vi "Multidimensional Array Example.vi"() -> ()   [LabVIEW 2015, in "MsgPack.lvlib"]
uses:
  MsgPack.lvlib
panel:
  out "1D Array - Recovered":dbl[](array[numeric]) format="%.2f"
  out "2D Array - Recovered":dbl[][](array[numeric]) format="%.2f"
  out "3D Array - Recovered":dbl[][][](array[numeric]) format="%.2f"
  in  "Seed":dbl
  out "3D Array Msgpack":string
  out "3D Error":errorcluster
  out "2D Array Msgpack":string
  out "2D Error":errorcluster
  out "1D Error":errorcluster
  out "1D Array Msgpack":string
  in  "Array Size":i32=1
  out "3D Array":dbl[][][](array[numeric]) format="%.2f"
  out "2D Array":dbl[][](array[numeric]) format="%.2f"
  out "1D Array":dbl[](array[numeric]) format="%.2f"
  # "This example shows how Multi-dimensional Arrays are serialized into a MsgPack Packet.\n\n1 - Adjust Seed value.\n2 - Change Seed datatype \n3 - Adjust Array Size\n\nNote:  The 2D and 3D Arrays are built from the smaller arrays with their superior dimension increased by 1."
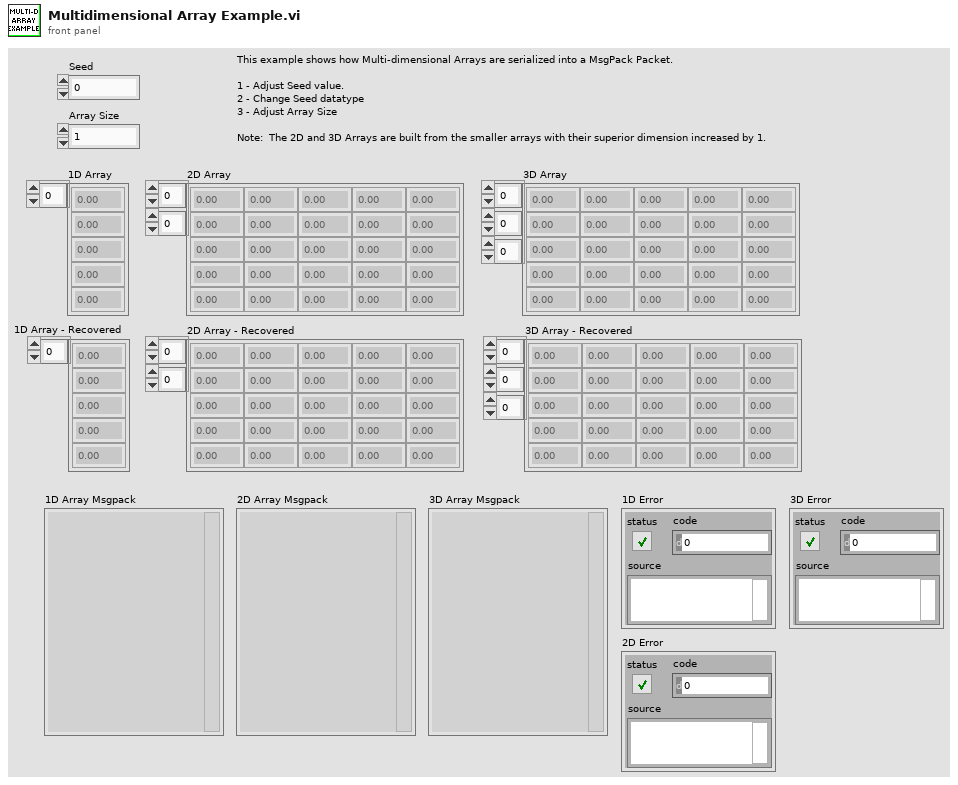
[diagram p1: front panel]
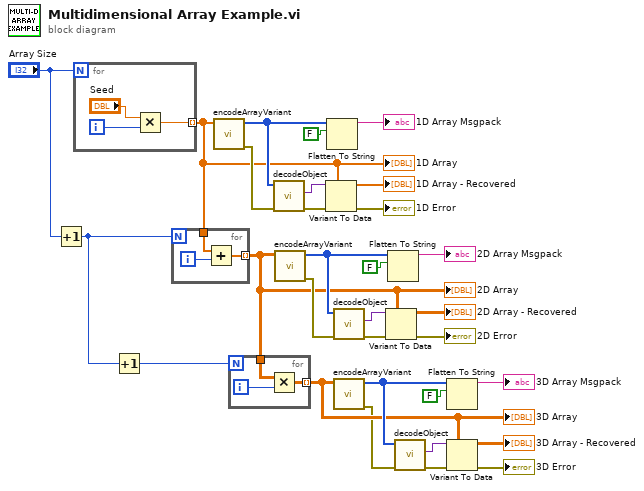
[diagram p0: block diagram]
diagram:
  n1 = Increment(x="Array Size") -> (x+1=w22:i32)
  n2 = for {
    N: "Array Size" -> [_]
    tunnel: [w32] -> w2 mode=indexing
    i -> [w33]
    n3 = Multiply(x="Seed", y=w33) -> (x*y=w32:dbl)
  }
  "1D Array" <- w2
  n4 = Increment(x=w22) -> (x+1=w25:i32)
  n5 = for {
    N: w22 -> [_]
    tunnel: w2 -> [w36]
    tunnel: [w34] -> w9 mode=indexing
    i -> [w35]
    n6 = Add(x=w36, y=w35) -> (x+y=w34:dbl[])
  }
  "2D Array" <- w9
  n7 = call "encodeArrayVariant.vi"("Variant"=w2) -> ("error out"=w3:errorcluster, "MessagePack"=w4:u8[])  [unwired: 9 in]
  n8 = for {
    N: w25 -> [_]
    tunnel: w9 -> [w39]
    tunnel: [w38] -> w18 mode=indexing
    i -> [w37]
    n9 = Multiply(x=w39, y=w37) -> (x*y=w38:dbl[][])
  }
  "3D Array" <- w18
  n10 = call "decodeObject.vi"("error in (no error)"=w3, "ByteArray"=w4) -> ("error out"=w7:errorcluster, "Variant"=w8:variant)  [unwired: 6 in, 2 out]
  n11 = call "encodeArrayVariant.vi"("Variant"=w9) -> ("error out"=w12:errorcluster, "MessagePack"=w13:u8[])  [unwired: 9 in]
  n12 = Variant To Data(error in=w7, type=w2, Variant=w8) -> (data=→"1D Array - Recovered":dbl[], error out=→"1D Error":errorcluster)
  n13 = Flatten To String(anything=w4, prepend array or string size? (T)=FALSE) -> (data string=→"1D Array Msgpack":string)  [unwired: 2 in, 2 out]
  n14 = call "decodeObject.vi"("error in (no error)"=w12, "ByteArray"=w13) -> ("error out"=w14:errorcluster, "Variant"=w1:variant)  [unwired: 6 in, 2 out]
  n15 = call "encodeArrayVariant.vi"("Variant"=w18) -> ("error out"=w16:errorcluster, "MessagePack"=w21:u8[])  [unwired: 9 in]
  n16 = Variant To Data(error in=w14, type=w9, Variant=w1) -> (data=→"2D Array - Recovered":dbl[][], error out=→"2D Error":errorcluster)
  n17 = Flatten To String(anything=w13, prepend array or string size? (T)=FALSE) -> (data string=→"2D Array Msgpack":string)  [unwired: 2 in, 2 out]
  n18 = call "decodeObject.vi"("error in (no error)"=w16, "ByteArray"=w21) -> ("error out"=w20:errorcluster, "Variant"=w19:variant)  [unwired: 6 in, 2 out]
  n19 = Flatten To String(anything=w21, prepend array or string size? (T)=FALSE) -> (data string=→"3D Array Msgpack":string)  [unwired: 2 in, 2 out]
  n20 = Variant To Data(error in=w20, type=w18, Variant=w19) -> (data=→"3D Array - Recovered":dbl[][][], error out=→"3D Error":errorcluster)
